vi "Command_Goto.vi"(0 "error in":errorcluster, 2 "Parameters":cluster{"Side":T1, "Desired Position":sgl}={"Side"=enum."left", "Desired Position"=100.0} {"Desired Position" min=0 max=100}, 3 "node":string) -> (1 "error out":errorcluster)   [LabVIEW 2014]
doc: "This will open or close the gripper to a specific position"
uses:
  ROS/Code/SubVIs/BaxterSide.ctl
  ROS/Code/Console/Servers/ServerSubs/TopicDef.ctl
  ROS/Code/SubVIs/_ROSDirection.ctl
panel:
  # "Gripper position is from [0.0-100.0] [close-open]"
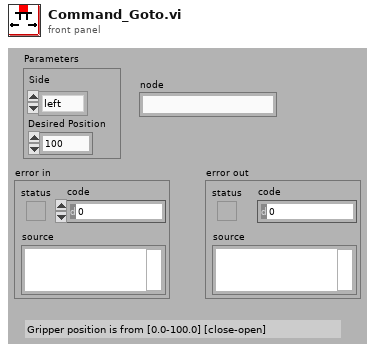
[diagram p1: front panel]
types:
  T1 = typedef "BaxterSide.ctl" = enum16{"left", "right"}
  T2 = typedef "TopicDef.ctl" = cluster{"Topic":string, "Type":string, "Action":T3, "Update (ms)":u16, "queue size":u16}
  T3 = typedef "_ROSDirection.ctl" = enum16{"Node", "Publisher", "Subscriber", "ServiceClient", "ServiceProvider"}
  T4 = enum16{"no_op", "set", "configure", "reboot", "reset", "calibrate", "clear_calibration", "prepare_to_grip", "grip", "release", "go", "stop"}
  T5 = typedef "_ROSControl.ctl" = cluster{"topic port":u16, "Node":string, "topic":string, "type":string, "node port":u16, "error ":errorcluster, "Direction":T3, "Update (ms)":u16, "FIFO size":u16}
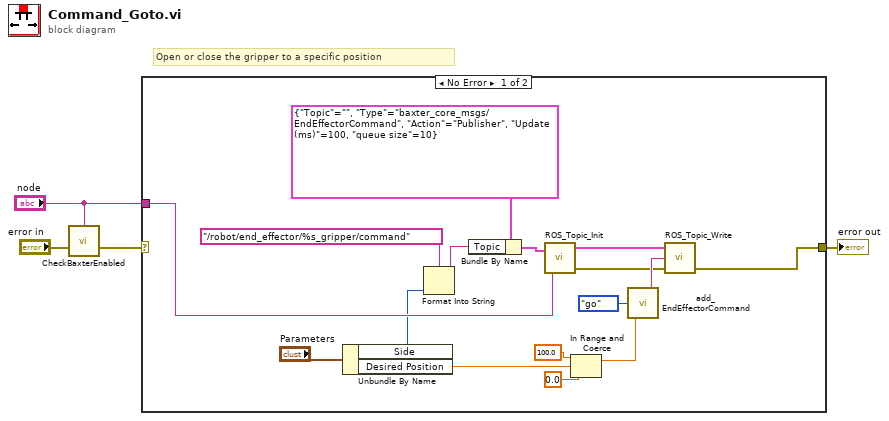
[diagram p0: block diagram]
diagram:
  # "Open or close the gripper to a specific position"
  n1 = call "CheckBaxterEnabled.vi"("error in"="error in", "node"="node") -> ("error out"=w2:errorcluster)  [unwired: 2 in]
  n2 = case shown="No Error" w2 {
    selector: w2 -> [_ w21]
    tunnel: [w8 w21] -> w4
    tunnel: "node" -> [w12 _]
    frame No Error {
      n3 = Unbundle By Name("Parameters") -> ("Side"=w6:T1, "Desired Position"=w5:sgl)
      n4 = Format Into String(format string="/robot/end_effector/%s_gripper/command" ("Topic"), w6) -> (resulting string=w14:string)  [unwired: 2 in, 1 out]
      n5 = Bundle By Name(cluster=T2 {"Topic"="", "Type"="baxter_core_msgs/EndEffectorCommand", "Action"=enum."Publisher", "Update (ms)"=100, "queue size"=10} ("Definitions"), "Topic"=w14) -> (w11:T2)
      n6 = call "ROS_Topic_Init.vi"("Definitions"=w11, "node"=w12) -> ("ROS out"=w20:T5, "error out"=w9:errorcluster)  [unwired: 1 in]
      n7 = In Range and Coerce(upper limit=sgl 100.0, x=w5, lower limit=sgl 0.0) -> (coerced(x)=w16:sgl)  [unwired: 1 out]
      n8 = call "add_EndEffectorCommand.vi"("Position"=w16, "Commands"=T4."go") -> ("msg out"=w10:string)  [unwired: 3 in]
      n9 = call "ROS_Topic_Write.vi"("error in (no error)"=w9, "Msg in"=w10, "ROS in"=w20) -> ("error out"=w8:errorcluster)  [unwired: 1 in, 1 out]
    }
    frame Error {
    }
  }
  "error out" <- w4
